vi "Create MQTT Client.vi"(5 "Client in":refnum<class "Client.lvclass">, 8 "error in (no error)":errorcluster, 10 "Connection Configuration":refnum<class "Connection.lvclass">, 11 "ID (empty:generate new)":string) -> (0 "error out":errorcluster, 3 "Client out":refnum<class "Client.lvclass">)   [LabVIEW 2013, in "MQTT Client.lvlib" / "Client.lvclass"]
uses:
  Client.lvclass
  MQTT_Connection/Connection/Connection.lvclass
  <vilib>/LabVIEW Open Source Project/MQTT Control Packets/Control Packets/CONNACK/Connect Return Code -- enum.ctl
  <vilib>/LabVIEW Open Source Project/MQTT Control Packets/Control Packets/PUBLISH/PUBLISH.lvclass
  MQTT_Base/Base Class/MQTT_Base.lvclass/MQTT_Base.ctl
  Client.lvclass/Client.ctl
  <vilib>/LabVIEW Open Source Project/Serializer/Serializer.FlattenedString/Serializer.FlattenedString.lvclass
  <vilib>/LabVIEW Open Source Project/Serializer/Serializer/Serializer.lvclass
  <vilib>/LabVIEW Open Source Project/MQTT Control Packets/Control Packets/ControlPacket/ControlPacket.lvclass
  <vilib>/LabVIEW Open Source Project/MQTT Control Packets/Control Packets/CONNACK/CONNACK.lvclass
  MQTT_Base/Base Class/MQTT_Base.lvclass
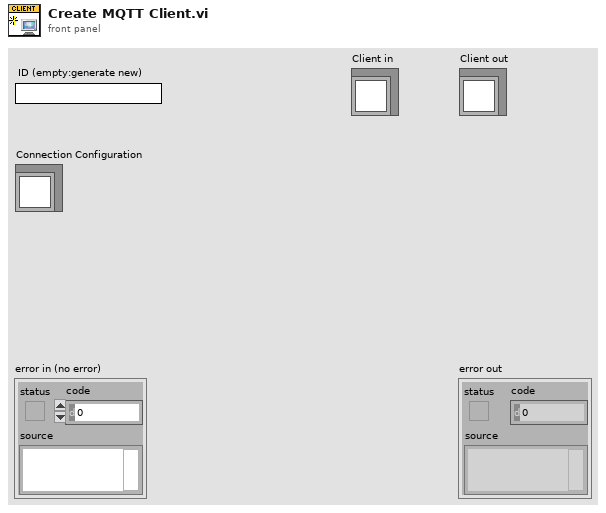
[diagram p1: front panel]
types:
  T1 = typedef "MQTT_Control_Packets.lvlib/CONNACK.lvclass/Connect Return Code -- enum.ctl" = enum16{"Connection accepted", "Unacceptable protocol version", "Identifier Rejected", "Server Unavailable", "Bad Username or Password", "Not Authorized"}
  T2 = cluster{"Connection Status":refnum<user-event>, "Connected":refnum<user-event>, "Application Message":refnum<user-event>}
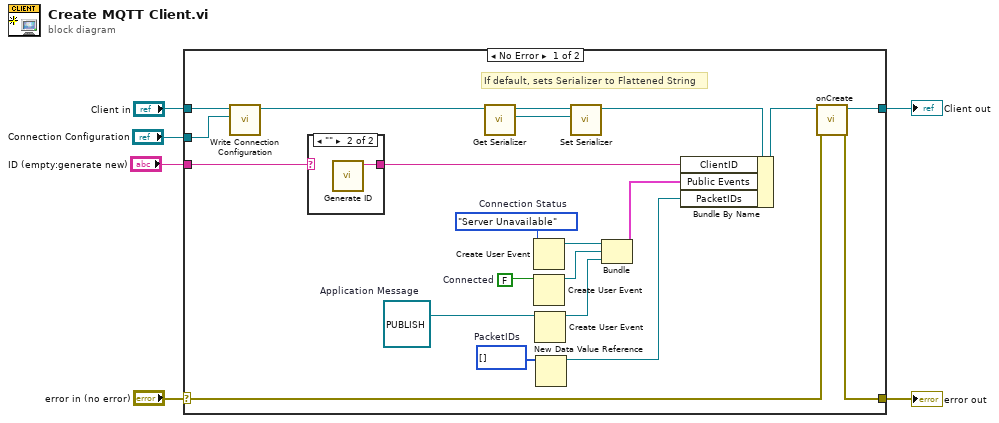
[diagram p0: block diagram]
diagram:
  n1 = case shown="No Error" "error in (no error)" {
    selector: "error in (no error)" -> [w23 w31]
    tunnel: [w22 w31] -> w2
    tunnel: [w24 w30] -> w3
    tunnel: "Client in" -> [w9 w30]
    tunnel: "ID (empty:generate new)" -> [w27 _]
    tunnel: "Connection Configuration" -> [w7 _]
    frame No Error {
      w14 = u16[] []  # PacketIDs
      w16 = refnum<class "PUBLISH.lvclass"> refnum  # Application Message
      w17 = FALSE  # Connected
      w19 = Connect_Return_Code_--_enum."Server Unavailable"  # Connection Status
      # "If default, sets Serializer to Flattened String"
      n2 = call "Write Connection Configuration.vi"("Connection Configuration"=w7, "MQTT_Base in"=w9) -> ("MQTT_Base out"=w8:refnum<class "Client.lvclass">)  [unwired: 8 in, 1 out]
      n3 = case shown="\"\"" w27 {
        selector: w27 -> [w28 _]
        tunnel: [w28 w29] -> w26
        frame Default {
        }
        frame "" {
          n4 = call <vilib>:"Generate ID.vi"() -> ("ID"=w29:string)  [unwired: 11 in]
        }
      }
      n5 = call "Get Serializer.vi"("MQTT_Base"=w8) -> ("Serializer"=w10:refnum<class "Serializer.lvclass">, "MQTT_Base out"=w12:refnum<class "Client.lvclass">)  [unwired: 8 in, 1 out]
      n6 = Create User Event(user event datatype=w19) -> (user event=w21:refnum<user-event>)  [unwired: 1 in, 1 out]
      n7 = Create User Event(user event datatype=w17) -> (user event=w18:refnum<user-event>)  [unwired: 1 in, 1 out]
      n8 = Create User Event(user event datatype=w16) -> (user event=w15:refnum<user-event>)  [unwired: 1 in, 1 out]
      n9 = New Data Value Reference(data value=w14) -> (data value reference=w13:refnum<data-value>)  [unwired: 1 in, 1 out]
      n10 = call "Set Serializer.vi"("Serializer (default: Flattened String)"=w10, "MQTT_Base"=w12) -> ("MQTT_Base out"=w11:refnum<class "Client.lvclass">)  [unwired: 8 in, 1 out]
      n11 = Bundle("Connection Status"=w21, "Connected"=w18, "Application Message"=w15) -> (w20:T2)  [unwired: 1 in]
      n12 = Bundle By Name(cluster=w11, "ClientID"=w26, "Public Events"=w20, "PacketIDs"=w13) -> (w25:refnum<class "Client.lvclass">)
      n13 = call-dynamic "onCreate.vi"("error in (no error)"=w23, "MQTT_Base in"=w25) -> ("error out"=w22:errorcluster, "MQTT_Base out"=w24:refnum<class "Client.lvclass">)  [unwired: 8 in]
    }
    frame Error {
    }
  }
  "error out" <- w2
  "Client out" <- w3
